vi "PDC_MRAWFileSaveOpen.vi"(6 "MaxFrameNum":i32, 7 "MRawBitDepth":u32, 8 "error in (no error)":errorcluster, 9 "FileName":string, 10 "ChildNo":u32, 11 "DeviceNo":u32) -> (0 "error out":errorcluster, 3 "ReturnValue":u32, 4 "ErrorCode":u32)   [LabVIEW 8.6]
doc: "This VI initializes the process to save recorded image data, on the device, to MRAW file."
uses:
  PDCLIB.dll
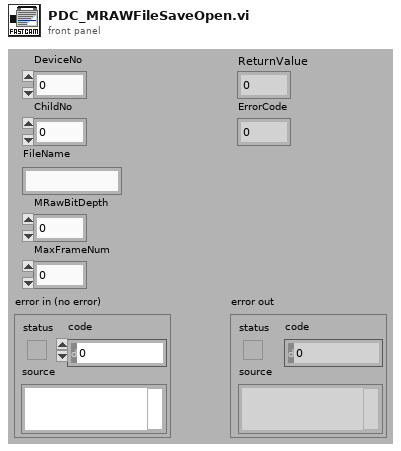
[diagram p1: front panel]
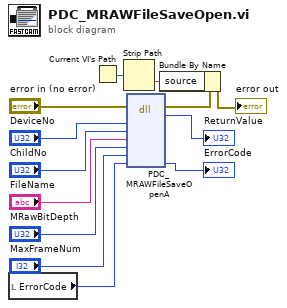
[diagram p0: block diagram]
diagram:
  n1 = local read "ErrorCode"() -> (w10:u32)
  n2 = Current VI's Path() -> (path=w3:path)
  n3 = Strip Path(path=w3) -> (name=w4:string)  [unwired: 1 out]
  n4 = dll-call lib="PDCLIB.dll" fn="PDC_MRAWFileSaveOpenA"(error in="error in (no error)", "nDeviceNo"="DeviceNo", "nChildNo"="ChildNo", "lpszFileName"="FileName", "nMRawBitDepth"="MRawBitDepth", "nMaxFrameNum"="MaxFrameNum", "pErrorCode"=w10) -> (error out=w2:errorcluster, "return type"=→"ReturnValue":u32, "pErrorCode"=→"ErrorCode":u32)  [unwired: 7 in, 1 out]
  n5 = Bundle By Name(cluster=w2, "source"=w4) -> (→"error out":errorcluster)
